vi "Get API Interface Info.vi"(8 "error in (no error)":errorcluster, 10 "CASE":string, 11 "CSM-Helper in":refnum<class "CSM-Helper.lvclass">) -> (0 "error out":errorcluster, 1 "Response":T1, 2 "Argument":T1, 3 "CSM-Helper out":refnum<class "CSM-Helper.lvclass">)   [LabVIEW 2020, in "CSM-Helper.lvclass"]
uses:
  CSM-Helper.lvclass
  Typedef/Def-Argument Info.ctl
  CSM-Helper.lvclass/CSM-Helper.ctl
  2ef4439d-e33a-454d-9680-145465e9d151.vi
  2ef4439d-e33a-454d-9680-145465e9d151.vi/eb2405bd-5b2e-436b-9bb3-692ecf4a9268.vi
  2ef4439d-e33a-454d-9680-145465e9d151.vi/c8ad12e3-5e6d-40e1-92e0-1426ef45ec41.vi
  2ef4439d-e33a-454d-9680-145465e9d151.vi/effcbc1a-e97c-42d4-b61f-d821de102707.vi
  48f19014-0606-45ab-83db-8268bac75835.vi
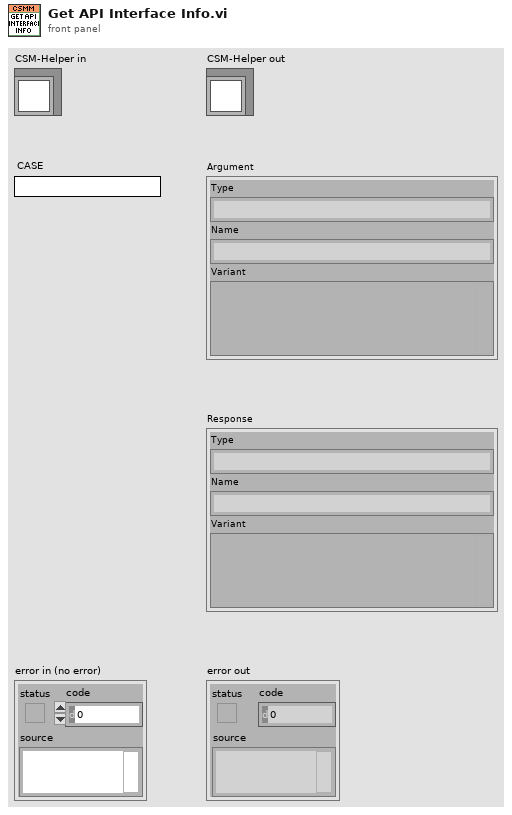
[diagram p1: front panel]
types:
  T1 = typedef "CSM-Helper.lvclass/Def-Argument Info.ctl" = cluster{"Type":string, "Name":string, "Variant":variant}
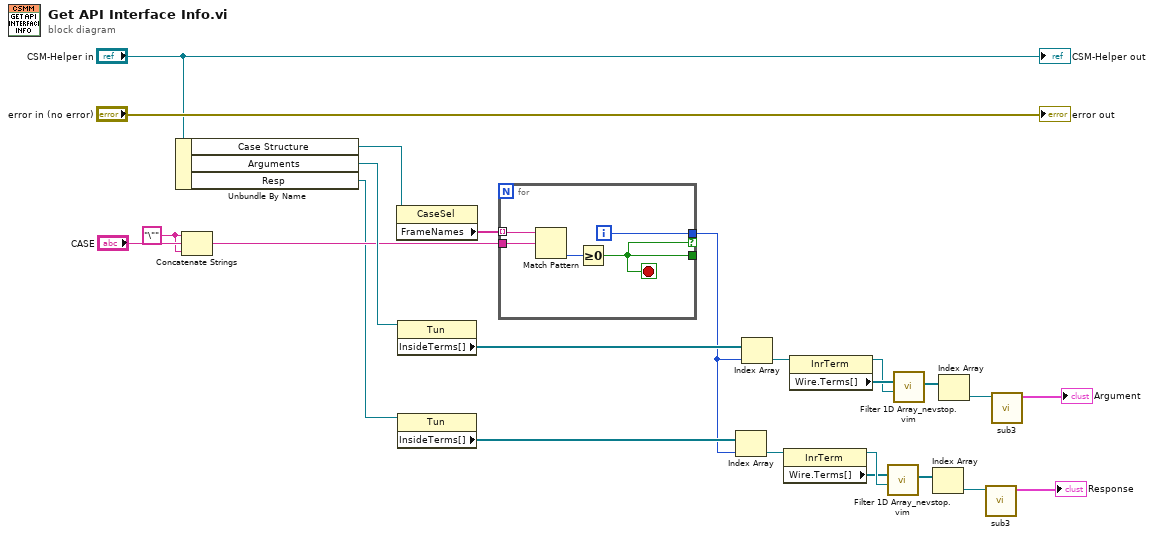
[diagram p0: block diagram]
diagram:
  w17 = "\"" ("string")
  n1 = Unbundle By Name("CSM-Helper in") -> ("Case Structure"=w22:refnum<vi>, "Arguments"=w21:refnum<vi>, "Resp"=w9:refnum<vi>)
  n2 = Concatenate Strings(w17, "CASE", w17) -> (w18:string)
  n3 = property class="CaseSel"(reference=w22) -> ("FrameNames"=w20:string[])  [unwired: 1 in, 2 out]
  n4 = property class="Tun"(reference=w21) -> ("InsideTerms[]"=w16:refnum<vi>[])  [unwired: 1 in, 2 out]
  n5 = property class="Tun"(reference=w9) -> ("InsideTerms[]"=w10:refnum<vi>[])  [unwired: 1 in, 2 out]
  n6 = for {
    tunnel: w20 -> [w29] mode=indexing
    tunnel: w18 -> [w28]
    tunnel: [w27] -> w8 if=w25
    tunnel: [w25] -> _
    i -> [w27]
    stop <- w25 stop-if-true
    n7 = Match Pattern(string=w29, regular expression=w28) -> (offset past match=w26:i32)  [unwired: 1 in, 3 out]
    n8 = Greater Or Equal To 0?(x=w26) -> (x >= 0?=w25:bool)
  }
  n9 = Index Array(array=w10, index=w8) -> (element=w3:refnum<vi>)
  n10 = Index Array(array=w16, index=w8) -> (element=w15:refnum<vi>)
  n11 = property class="InrTerm"(reference=w3) -> (reference out=w5:refnum<vi>, "Wire.Terms[]"=w4:refnum<vi>[])  [unwired: 1 in, 1 out]
  n12 = property class="InrTerm"(reference=w15) -> (reference out=w13:refnum<vi>, "Wire.Terms[]"=w14:refnum<vi>[])  [unwired: 1 in, 1 out]
  n13 = call "Filter 1D Array_nevstop.vim"("items to filter"=w5, "array"=w4) -> ("filtered array"=w6:refnum<vi>[])  [unwired: 4 in, 1 out]
  n14 = call "Filter 1D Array_nevstop.vim"("items to filter"=w13, "array"=w14) -> ("filtered array"=w12:refnum<vi>[])  [unwired: 4 in, 1 out]
  n15 = Index Array(array=w6) -> (element=w1:refnum<vi>)  [unwired: 1 in]
  n16 = Index Array(array=w12) -> (element=w11:refnum<vi>)  [unwired: 1 in]
  n17 = call "sub3.vi"("Terminal in"=w1) -> ("Argument"=→"Response":T1)  [unwired: 10 in]
  n18 = call "sub3.vi"("Terminal in"=w11) -> ("Argument"=→"Argument":T1)  [unwired: 10 in]
  "error out" <- "error in (no error)"
  "CSM-Helper out" <- "CSM-Helper in"
